vi "Insight_Dialog_OPC.vi"(1 "canceled":bool, 8 "error in (no error)":errorcluster, 11 "telnet connection":T1) -> (0 "error out":errorcluster, 2 "seconds elapsed":dbl, 3 "telnet  connection out":T1)   [LabVIEW 2015]
uses:
  Telnet Session.ctl
panel:
  out "abort complete":bool
  out "stop":bool
  in  "Tab Control":enum32{"Waiting", "Aborting"}(tab)
  out "Waiting Indicator":cluster{u8, u8}(slide)={0, 49} caption="Search Indicator" scale=0.0..100.0
  out "Aborting Indicator":cluster{u8, u8}(slide)={0, 49} caption="Search Indicator" scale=0.0..100.0
  # "Waiting for operation to complete..."
  # "Waiting for operation to abort..."
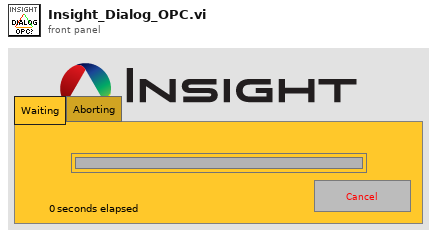
[diagram p1: front panel]
types:
  T1 = typedef "Telnet Session.ctl" = refnum<k1>
  T2 = enum32{"Invalid", "Default", "Floating", "Floating/Auto-Hide", "Modal"}
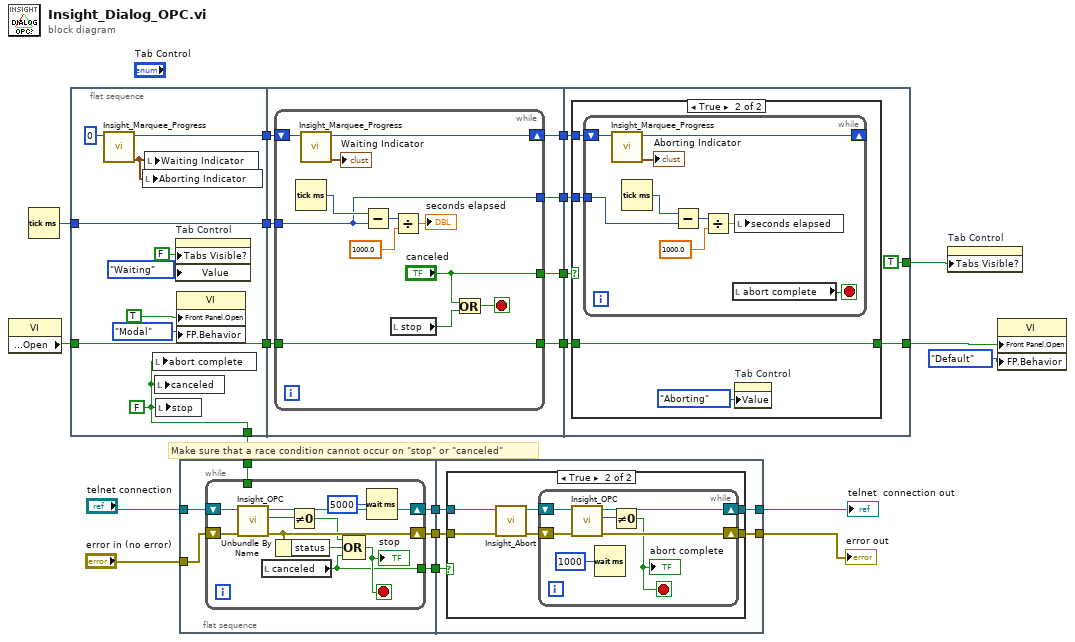
[diagram p0: block diagram]
diagram:
  # "Make sure that a race condition cannot occur on \"stop\" or \"canceled\""
  n1 = property class="VI"() -> ("Front Panel.Open"=w14:bool)  [unwired: 2 in, 2 out]
  n2 = Tick Count (ms)() -> (millisecond timer value=w18:u32)
  n3 = flat-sequence {
    tunnel: [w29] -> w20
    tunnel: [w28] -> w19
    tunnel: w18 -> [w28]
    tunnel: [w27] -> w15
    tunnel: w14 -> [w27]
    tunnel: [w21] -> w9
    tunnel: w20 -> [w37]
    tunnel: w19 -> [w36]
    tunnel: w15 -> [w34]
    tunnel: [w35] -> w8
    tunnel: [w33] -> w7
    tunnel: [w32] -> w6
    tunnel: [w31] -> w5
    tunnel: [w53] -> w16
    tunnel: w8 -> [w52]
    tunnel: w7 -> [w55]
    tunnel: w6 -> [w54]
    tunnel: w5 -> [w51]
    tunnel: [TRUE ("Tabs Visible?")] -> w1
    frame #0 {
      w21 = FALSE ("stop")
      n4 = call "Insight_Marquee_Progress.vi"("x"=u8 0) -> ("Progress Indicator"=w22:cluster{u8, u8}, "x (out)"=w29:u8)  [unwired: 9 in]
      n5 = local write "Aborting Indicator"(w22) -> ()
      n6 = local write "Waiting Indicator"(w22) -> ()
      n7 = local write "abort complete"(w21) -> ()
      n8 = local write "canceled"(w21) -> ()
      n9 = local write "stop"(w21) -> ()
      n10 = property on="Tab Control" class="TabCtl (strict)"("Tabs Visible?"=FALSE, "Value"=enum32{"Waiting", "Aborting"}."Waiting" ("Tab Control")) -> ()  [unwired: 2 in, 2 out]
      n11 = property class="VI"("Front Panel.Open"=TRUE ("Front Panel Window:Open"), "FP.Behavior"=T2."Modal" ("Front Panel Window:Behavior")) -> ()  [unwired: 2 in, 2 out]
    }
    frame #1 {
      n12 = while {
        shift-right: [w47] -> w33
        shift-left: w37 -> [w49]
        tunnel: w36 -> [w38]
        tunnel: [w41] -> w35
        tunnel: w34 -> [w41]
        tunnel: ["canceled"] -> w32
        tunnel: [w38] -> w31
        stop <- w42 stop-if-true
        n13 = Tick Count (ms)() -> (millisecond timer value=w44:u32)
        n14 = call "Insight_Marquee_Progress.vi"("x"=w49) -> ("Progress Indicator"=→"Waiting Indicator":cluster{u8, u8}, "x (out)"=w47:u8)  [unwired: 9 in]
        n15 = Subtract(x=w44, y=w38) -> (x-y=w45:u32)
        n16 = local read "stop"() -> (w40:bool)
        n17 = Divide(x=w45, y=1000.0) -> (x/y=→"seconds elapsed":dbl)
        n18 = Or(x="canceled", y=w40) -> (x .or. y?=w42:bool)
      }
    }
    frame #2 {
      n19 = case shown="True" w54 {
        tunnel: w55 -> [_ w60]
        tunnel: [w56 w57] -> w53
        tunnel: w52 -> [w56 w57]
        tunnel: w51 -> [_ w59]
        frame False {
        }
        frame True {
          n20 = while {
            shift-right: [w68] -> _
            shift-left: w60 -> [w69]
            tunnel: w59 -> [w64]
            stop <- w61 stop-if-true
            n21 = call "Insight_Marquee_Progress.vi"("x"=w69) -> ("Progress Indicator"=→"Aborting Indicator":cluster{u8, u8}, "x (out)"=w68:u8)  [unwired: 9 in]
            n22 = Tick Count (ms)() -> (millisecond timer value=w65:u32)
            n23 = Subtract(x=w65, y=w64) -> (x-y=w66:u32)
            n24 = Divide(x=w66, y=1000.0) -> (x/y=w63:dbl)
            n25 = local read "abort complete"() -> (w61:bool)
            n26 = local write "seconds elapsed"(w63) -> ()
          }
          n27 = property on="Tab Control" class="TabCtl (strict)"("Value"=enum32{"Waiting", "Aborting"}."Aborting" ("Tab Control")) -> ()  [unwired: 2 in, 2 out]
        }
      }
    }
  }
  n28 = flat-sequence {
    tunnel: "telnet connection" -> [w75]
    tunnel: "error in (no error)" -> [w74]
    tunnel: w9 -> [w71]
    tunnel: [w73] -> w4
    tunnel: [w72] -> w3
    tunnel: [w70] -> w2
    tunnel: [w87] -> w10
    tunnel: [w89] -> w11
    tunnel: w4 -> [w90]
    tunnel: w3 -> [w88]
    tunnel: w2 -> [w91]
    frame #0 {
      n29 = while {
        shift-right: [w83] -> w73
        shift-left: w75 -> [w85]
        shift-right: [w80] -> w72
        shift-left: w74 -> [w84]
        tunnel: [w81] -> _
        tunnel: w71 -> [w81]
        tunnel: [w76] -> w70
        stop <- w78 stop-if-true
        n30 = call "Insight_OPC.vi"("error in (no error)"=w84, "telnet connection"=w85) -> ("error out"=w80:errorcluster, "OPC Bit value (1=Idle)"=w86:u32, "telnet  connection out"=w83:T1)  [unwired: 6 in, 1 out]
        n31 = local read "canceled"() -> (w76:bool)
        n32 = Unbundle By Name(w80) -> ("status"=w77:bool)
        n33 = Not Equal To 0?(x=w86) -> (x != 0?=w79:bool)
        n34 = Compound Arithmetic op=OR(w79, w77, w76) -> (w78:bool)
        "stop" <- w78
        n35 = Wait (ms)(milliseconds to wait=u32 5000) -> ()  [unwired: 1 out]
      }
    }
    frame #1 {
      n36 = case shown="True" w91 {
        tunnel: w90 -> [w93 w99]
        tunnel: [w93 w95] -> w89
        tunnel: w88 -> [w92 w98]
        tunnel: [w92 w94] -> w87
        frame False {
        }
        frame True {
          n37 = call "Insight_Abort.vi"("error in (no error)"=w98, "telnet connection"=w99) -> ("error out"=w96:errorcluster, "telnet  connection out"=w97:T1)  [unwired: 7 in, 1 out]
          n38 = while {
            shift-right: [w103] -> w95
            shift-left: w97 -> [w106]
            shift-right: [w104] -> w94
            shift-left: w96 -> [w105]
            stop <- w101 stop-if-true
            n39 = call "Insight_OPC.vi"("error in (no error)"=w105, "telnet connection"=w106) -> ("error out"=w104:errorcluster, "OPC Bit value (1=Idle)"=w102:u32, "telnet  connection out"=w103:T1)  [unwired: 6 in, 1 out]
            n40 = Wait (ms)(milliseconds to wait=u32 1000) -> ()  [unwired: 1 out]
            n41 = Not Equal To 0?(x=w102) -> (x != 0?=w101:bool)
            "abort complete" <- w101
          }
        }
      }
    }
  }
  n42 = property on="Tab Control" class="TabCtl (strict)"("Tabs Visible?"=w1) -> ()  [unwired: 2 in, 2 out]
  n43 = property class="VI"("Front Panel.Open"=w16, "FP.Behavior"=T2."Default" ("Front Panel Window:Behavior")) -> ()  [unwired: 2 in, 2 out]
  "telnet  connection out" <- w11
  "error out" <- w10
